vi "SMO.ByRefWithEvents.Process.vi"(8 "error in (no error)":errorcluster, 11 "SMO.ByRefWithEvents in":refnum<class "SMO.ByRefWithEvents.lvclass">) -> (0 "error out":errorcluster)   [LabVIEW 2013, in "SMO.ByRefWithEvents.lvclass"]
uses:
  SMO.ByRefWithEvents.lvclass
  <vilib>/JKI/JKI SMO/SMO/SMO.lvclass
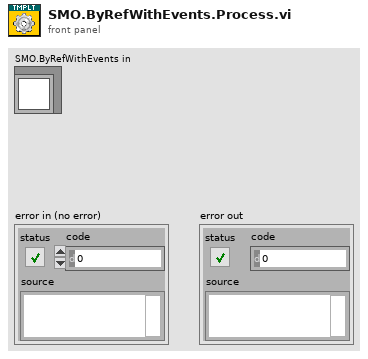
[diagram p1: front panel]
types:
  T1 = enum32{"invalid app kind", "Development System", "Run Time System", "Student Edition", "Embedded LabVIEW", "Evaluation", "Custom"}
  T2 = cluster{"Current VI Reference":refnum<vi>, "Close Panel on Exit?":bool, "error":errorcluster, "Standalone":bool}
  T3 = enum32{"Invalid", "Standard", "Closed", "Hidden", "Minimized", "Maximized"}
  T4 = cluster{"Core":cluster{"Current VI Reference":refnum<vi>, "Close Panel on Exit?":bool, "error":errorcluster, "Standalone":bool}, "Self Reference":refnum<class "SMO.ByRefWithEvents.lvclass">, "Your string data":string}
  T5 = typedef "SMO.lvclass/SMOState --Enum.ctl" = enum16{"unknown", "Created", "Started", "Stopped"}
  T6 = typedef "SMO.lvclass/Protected Events.ctl" = cluster{"StopProcesses":refnum<user-event>, "AbortProcesses":refnum<user-event>, "Config Changed":refnum<user-event>}
  T7 = typedef "SMO.ByRefWithEvents.lvclass/ProtectedEvents--Cluster.ctl" = cluster{"API_Template":refnum<user-event>}
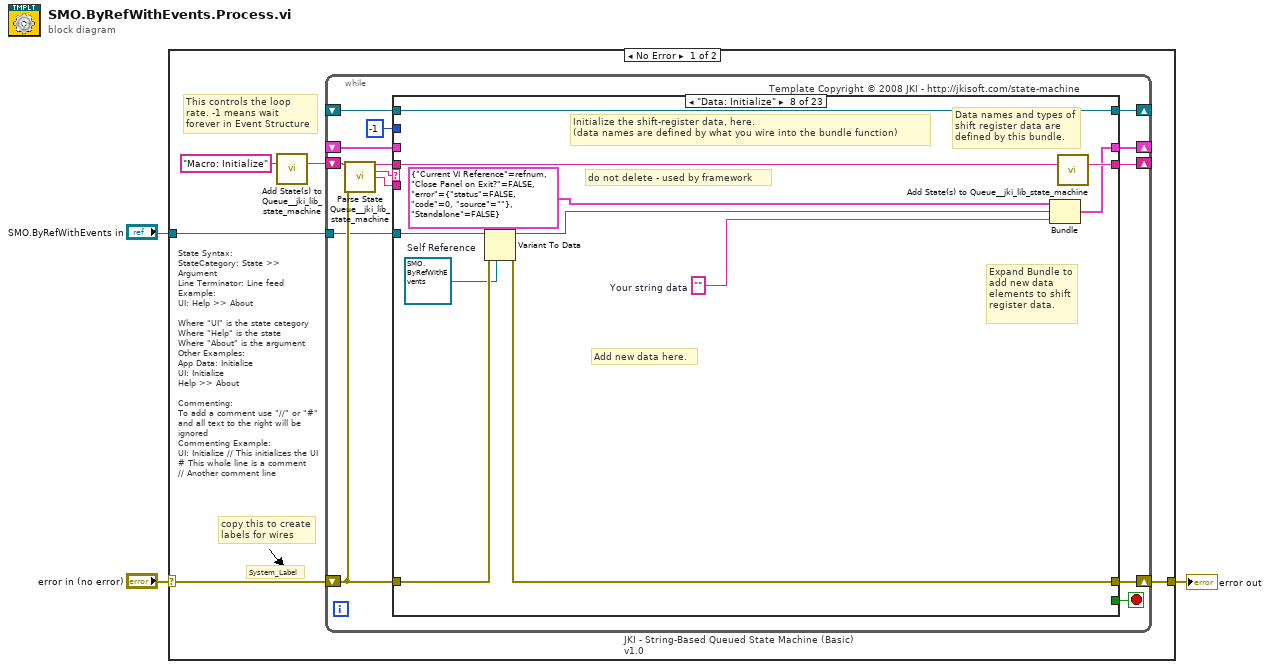
[diagram p0: block diagram]
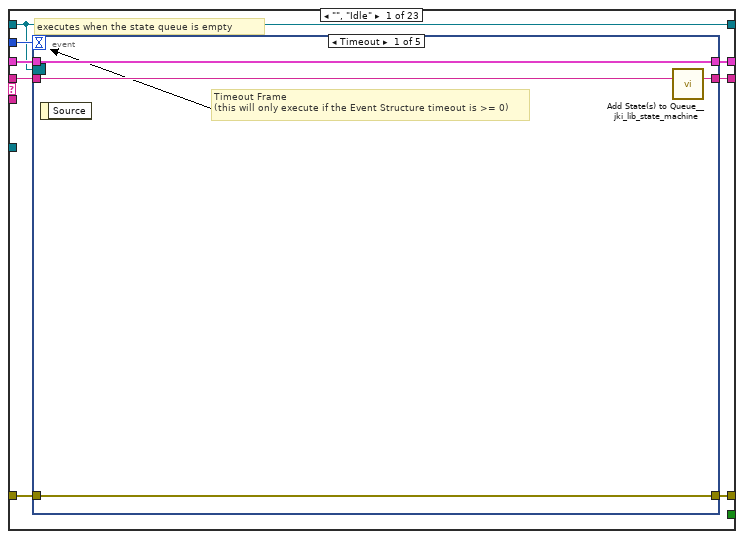
[diagram p2: hidden frame]
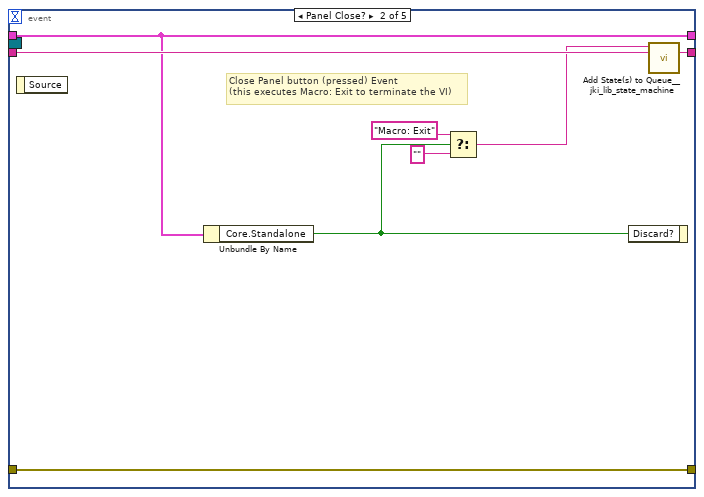
[diagram p3: hidden frame]
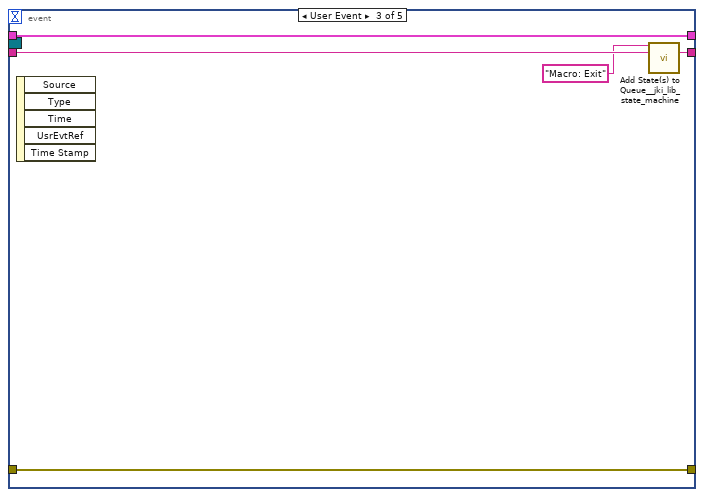
[diagram p4: hidden frame]
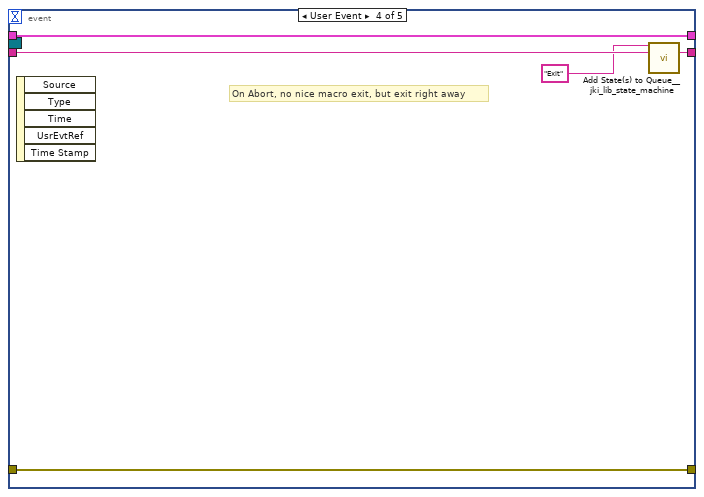
[diagram p5: hidden frame]
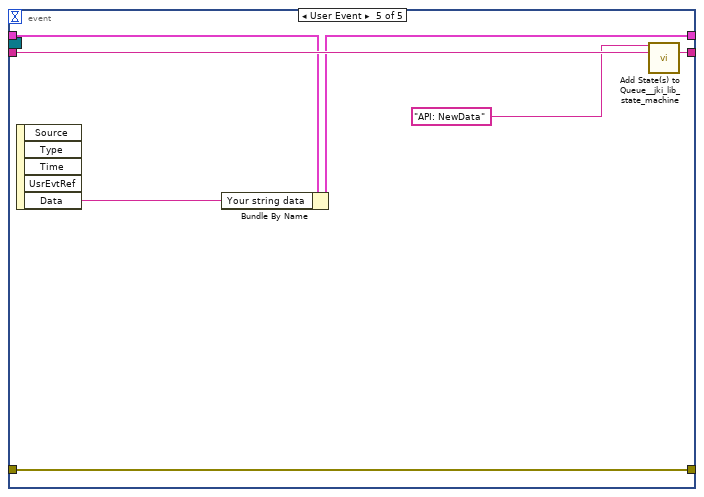
[diagram p6: hidden frame]
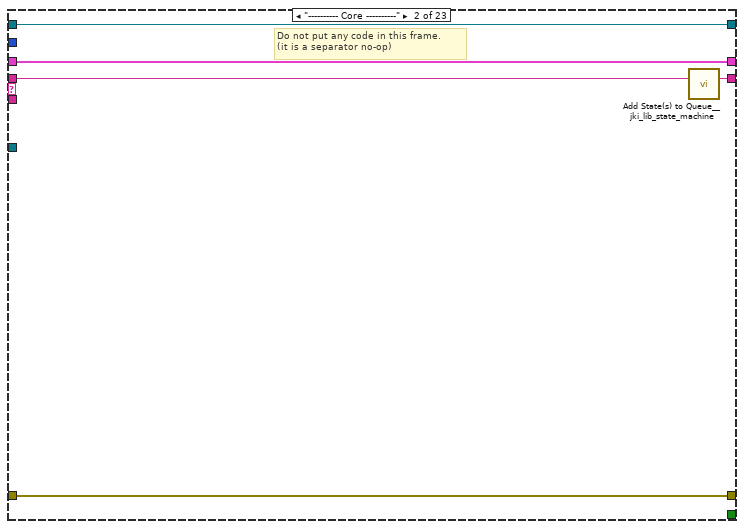
[diagram p7: hidden frame]
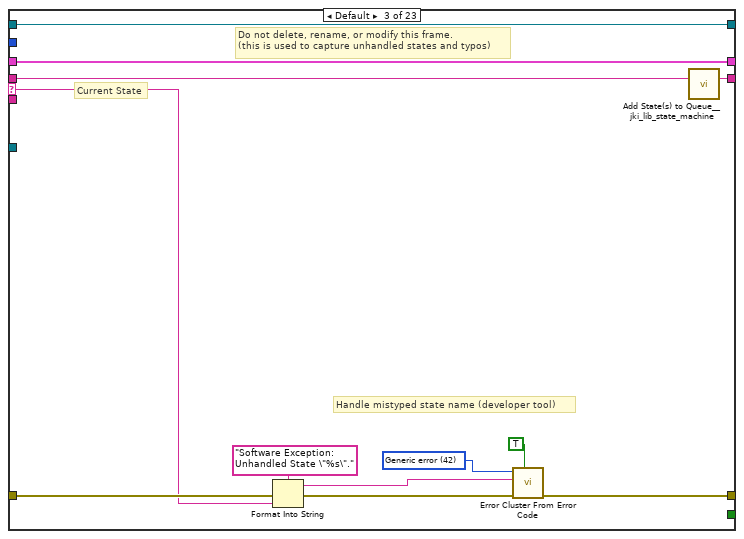
[diagram p8: hidden frame]
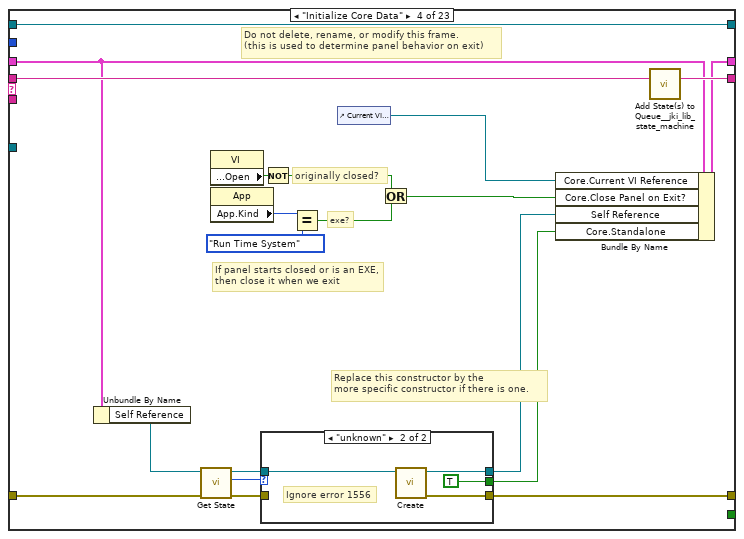
[diagram p9: hidden frame]
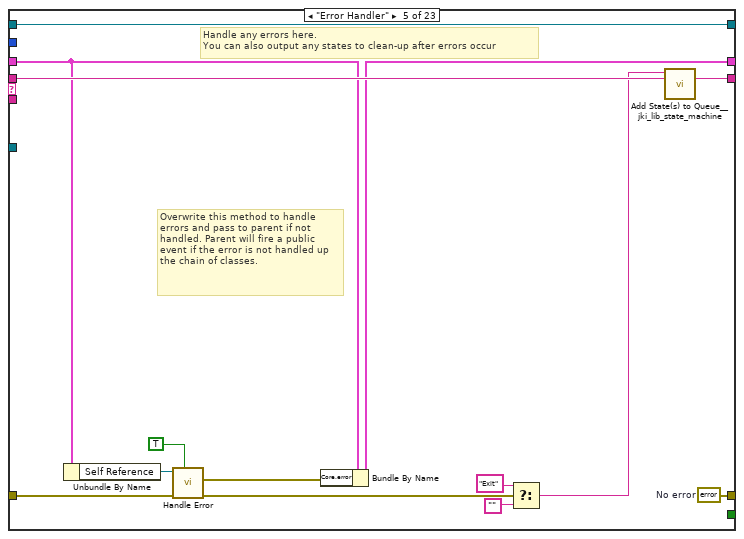
[diagram p11: hidden frame]
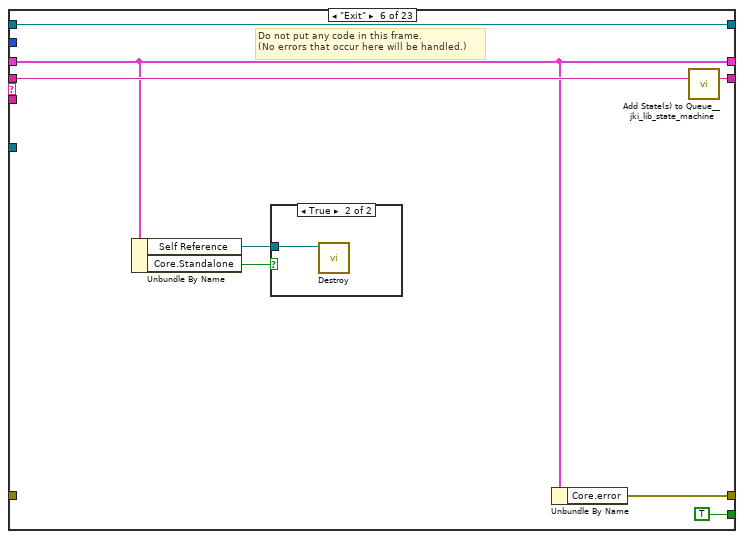
[diagram p12: hidden frame]
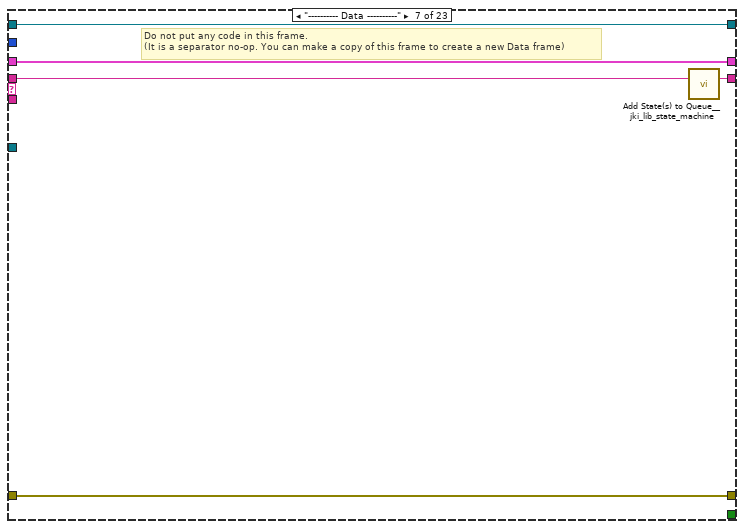
[diagram p14: hidden frame]
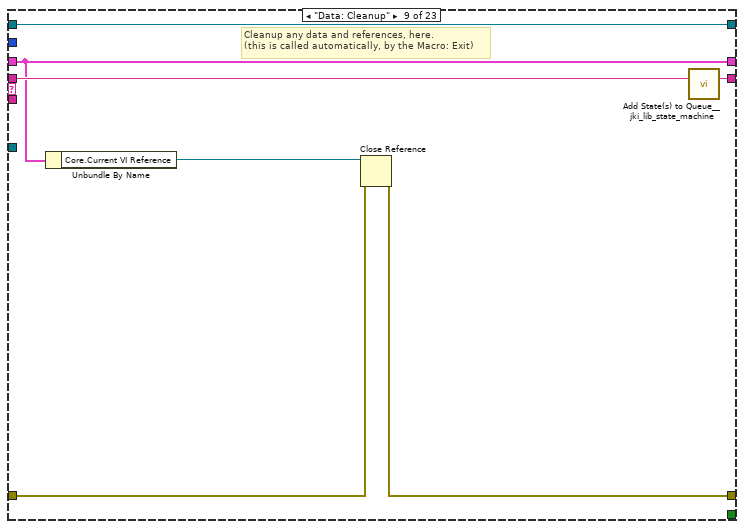
[diagram p15: hidden frame]
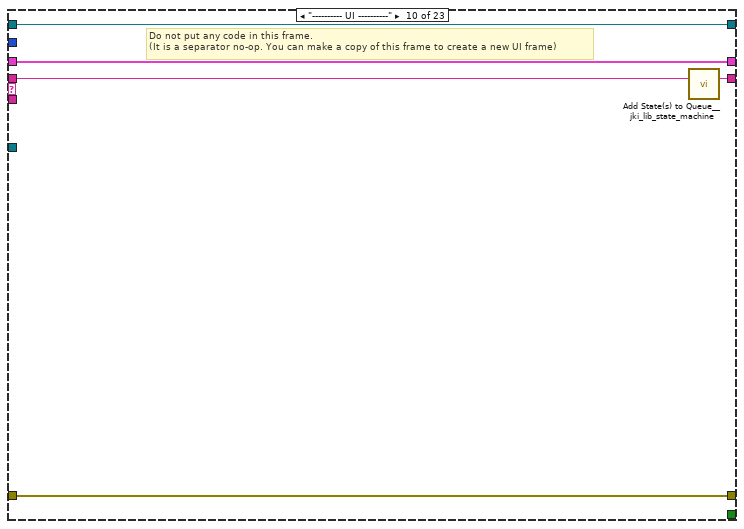
[diagram p16: hidden frame]
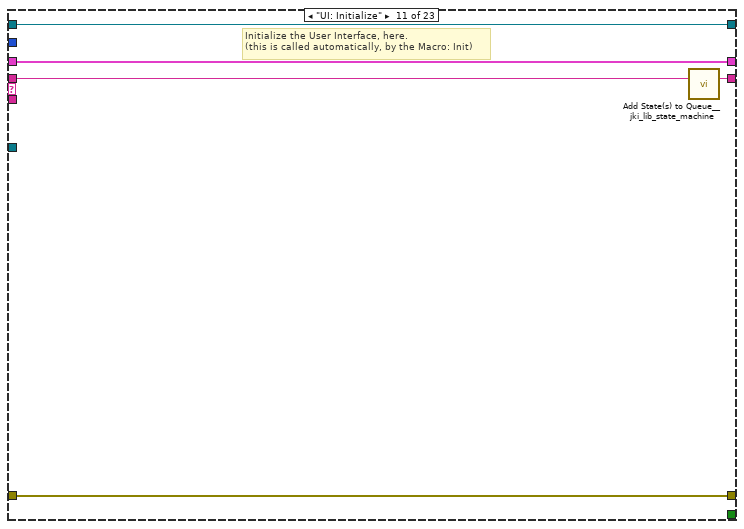
[diagram p17: hidden frame]
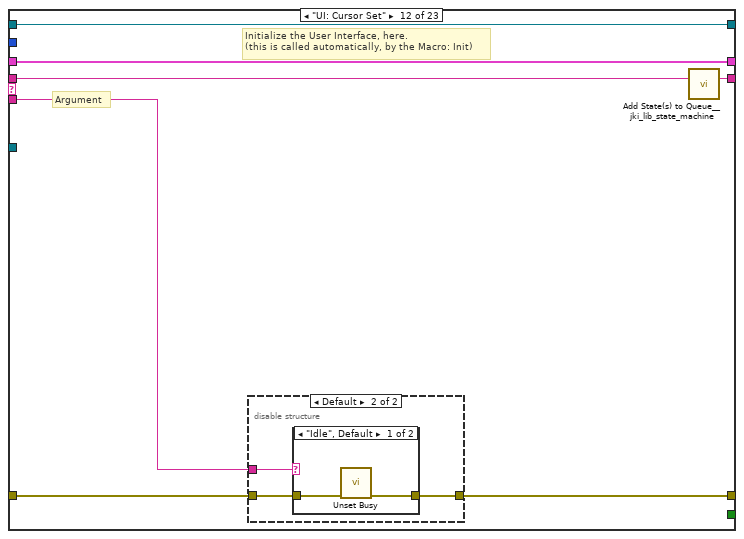
[diagram p18: hidden frame]
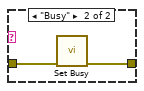
[diagram p20: hidden frame]
diagram:
  n1 = case shown="No Error" "error in (no error)" {
    selector: "error in (no error)" -> [w5 w290]
    tunnel: "SMO.ByRefWithEvents in" -> [w6 _]
    tunnel: [w4 w290] -> w3
    frame No Error {
      # "State Syntax:\nStateCategory: State >> Argument\nLine Terminator: Line feed\nExample:\nUI: Help >> About\n\nWhere \"UI\" is the state category\nWhere \"Help\" is the state\nWhere \"About\" is the argument\nOther Examples:\nApp Data: Initialize\nUI: Initialize\nHelp >> About\n\nCommenting:\nTo add a comment use \"//\" or \"#\" and all text to the right will be ignored\nCommenting Example:\nUI: Initialize // This initializes the UI\n# This whole line is a comment\n// Another comment line"
      # "copy this to create labels for wires"
      # "This controls the loop rate. -1 means wait forever in Event Structure"
      # "System_Label"
      n2 = call <vilib>:"Add State(s) to Queue__jki_lib_state_machine.vi"("State(s) in (\"\")"="Macro: Initialize") -> ("States Out"=w8:string)  [unwired: 14 in]
      n3 = while "JKI - String-Based Queued State Machine (Basic) v1.0" {
        shift-right: [w15] -> _
        shift-left: _ -> [w14]
        shift-right: [w18] -> w4
        shift-left: w5 -> [w12]
        shift-right: [w17] -> _
        shift-left: w8 -> [w19]
        tunnel: w6 -> [w11]
        shift-right: [w10] -> _
        shift-left: _ -> [w9]
        stop <- w16 stop-if-true
        # "Template Copyright © 2008 JKI - http://jkisoft.com/state-machine"
        n4 = call <vilib>:"Parse State Queue__jki_lib_state_machine.vi"("State Queue"=w19, "Error In (no error)"=w12) -> ("Remaining States"=w21:string, "Current State"=w22:string, "Arguments"=w20:string)  [unwired: 11 in]
        n5 = case shown="\"Data: Initialize\"" w22 {
          selector: w22 -> [_ _ w66 _ _ _ _ _ _ _ _ _ _ _ _ _ _ _ _ _ _ _ _]
          tunnel: w21 -> [w30 w64 w70 w96 w116 w124 w130 w141 w148 w153 w158 w165 w181 w213 w219 w230 w235 w244 w257 w270 w276 w281 w289]
          tunnel: w20 -> [_ _ _ _ _ _ _ _ _ _ _ w159 w175 _ _ _ _ _ _ _ _ _ _]
          tunnel: w14 -> [w28 w61 w68 w80 w105 w117 w127 _ w143 w150 w156 w163 w177 w210 w215 w221 w232 w241 w254 w268 w274 w279 w286]
          tunnel: [w27 w62 w72 w79 w107 w120 w128 w136 w144 w151 w155 w160 w178 w211 w217 w228 w233 w238 w255 w258 w272 w277 w282] -> w18
          tunnel: w12 -> [w26 w62 w71 w81 w112 _ w128 w137 w145 w151 w155 w161 w179 w211 w217 w228 w233 w239 w255 w262 w272 w277 w283]
          tunnel: [w29 w63 w69 w95 w115 w123 w129 w140 w147 w152 w157 w164 w180 w212 w218 w229 w234 w243 w256 w269 w275 w280 w288] -> w17
          tunnel: [_ _ _ _ _ TRUE _ _ _ _ _ _ _ _ _ _ _ _ _ _ _ _ _] -> w16
          tunnel: [w25 w61 w68 w94 w104 w117 w127 w139 w143 w150 w156 w163 w177 w210 w215 w221 w232 w241 w254 w268 w274 w279 w286] -> w15
          tunnel: -1 ("Timeout") -> [w24 _ _ _ _ _ _ _ _ _ _ _ _ _ _ _ _ _ _ _ _ _ _]
          tunnel: w11 -> [_ _ _ _ _ _ _ w134 _ _ _ _ _ _ _ _ _ _ _ _ _ _ _]
          tunnel: [w23 w60 w65 w87 w114 w121 w126 w132 w142 w149 w154 w162 w174 w209 w216 w222 w231 w242 w253 w267 w273 w278 w287] -> w10
          tunnel: w9 -> [w23 w60 w65 w87 w114 w121 w126 w132 w142 w149 w154 w162 w174 w209 w216 w222 w231 w242 w253 _ w273 w278 w287]
          frame "", "Idle" {
            # "executes when the state queue is empty"
            n6 = event shown="[0] Timeout" {
              selector: w23 -> [_ _ _ _ _]
              dyn-events: _ -> [_ _ _ _ _]
              timeout: w24 -> [_ _ _ _ _]
              tunnel: w30 -> [w34 w42 w47 w52 w59]
              tunnel: [w33 w41 w46 w51 w58] -> w29
              tunnel: w28 -> [w31 w37 w44 w49 w55]
              tunnel: [w32 w40 w45 w50 w57] -> w27
              tunnel: w26 -> [w32 w40 w45 w50 w57]
              tunnel: [w31 w37 w44 w49 w54] -> w25
              event Timeout {
                # "Timeout Frame\n(this will only execute if the Event Structure timeout is >= 0)"
                n7 = event-data() -> ()  [unwired: 1 in, 1 out]
                n8 = call <vilib>:"Add State(s) to Queue__jki_lib_state_machine.vi"("State(s) in (\"\")"=w34) -> ("States Out"=w33:string)  [unwired: 14 in]
              }
              event Panel Close? {
                # "Close Panel button (pressed) Event\n(this executes Macro: Exit to terminate the VI)"
                n9 = event-data() -> ()  [unwired: 1 in, 1 out]
                n10 = Unbundle By Name(w37) -> ("Core.Standalone"=w36:bool)
                n11 = Select(t="Macro: Exit", s=w36, f="") -> (s? t:f=w35:string)
                n12 = event-data("Discard?"=w36) -> ()  [unwired: 1 in, 1 out]
                n13 = call <vilib>:"Add State(s) to Queue__jki_lib_state_machine.vi"("State(s) in Front (\"\")"=w35, "State(s) in (\"\")"=w42) -> ("States Out"=w41:string)  [unwired: 13 in]
              }
              event User Event {
                n14 = event-data() -> ()  [unwired: 1 in, 5 out]
                n15 = call <vilib>:"Add State(s) to Queue__jki_lib_state_machine.vi"("State(s) in Front (\"\")"="Macro: Exit", "State(s) in (\"\")"=w47) -> ("States Out"=w46:string)  [unwired: 13 in]
              }
              event User Event {
                # "On Abort, no nice macro exit, but exit right away"
                n16 = event-data() -> ()  [unwired: 1 in, 5 out]
                n17 = call <vilib>:"Add State(s) to Queue__jki_lib_state_machine.vi"("State(s) in Front (\"\")"="Exit", "State(s) in (\"\")"=w52) -> ("States Out"=w51:string)  [unwired: 13 in]
              }
              event User Event {
                n18 = event-data() -> ("Data"=w56:string)  [unwired: 1 in, 4 out]
                n19 = Bundle By Name(cluster=w55, "Your string data"=w56) -> (w54:T4)
                n20 = call <vilib>:"Add State(s) to Queue__jki_lib_state_machine.vi"("State(s) in Front (\"\")"="API: NewData", "State(s) in (\"\")"=w59) -> ("States Out"=w58:string)  [unwired: 13 in]
              }
            }
          }
          frame "---------- Core ----------" {
            # "Do not put any code in this frame.\n(it is a separator no-op)"
            n21 = call <vilib>:"Add State(s) to Queue__jki_lib_state_machine.vi"("State(s) in (\"\")"=w64) -> ("States Out"=w63:string)  [unwired: 14 in]
          }
          frame Default {
            w75 = 42 items=["No error", "Argument error", "Memory is full", "Out of zone", "End of file", "File already open", "Generic file I/O error", "File not found", "File permission error", "Disk is full", "Duplicate path", "Too many files open", "System feature not enabled", "Resource file not found", "Cannot add resource", "Resource not found", "Image not found", "Image memory error", "Pen does not exist", "Config type invalid", "Config token not found", "Config parse error", "Config memory error", "Bad external code format", "Bad external code offset", "External code not present", "Null window", "Destroy window error", "Null menu", "Print aborted", "Bad print record", "Print driver error", "Windows error during printing", "Memory error during printing", "Print dialog error", "Generic print error", "Invalid device refnum", "Device not found", "Device parameter error", "Device unit error", "Cannot open device", "Device call aborted", "Generic error", "Cancelled by user", "Object ID too low", "Object ID too high", "Object not in heap", "Unknown heap", "Unknown object (invalid DefProc)", "Unknown object (DefProc not in table)", "Message out of range", "Invalid (null) method", "Unknown message", "Manager call not supported", "Bad address", "Network operation in progress", "Network operation timed out", "Connection is busy", "Network attribute not supported", "Network error", "Address in use", "System out of memory", "Connection aborted", "Connection refused", "Not connected", "Already connected", "Connection closed", "Initialization error (interapplication manager)", "Bad occurrence", "Wait on unbound occurrence handler", "Occurrence queue overflow", "Datalog type conflict", "Unused", "Unrecognized type (interapplication manager)", "Memory corrupt", "Failed to make temporary DLL", "Old CIN version", "Drag socket not found", "Failed to load drop-object", "Failed to register OLE object", "Failed to release OLE object", "Format specifier type mismatch", "Unknown format specifier", "Too few format specifiers", "Too many format specifiers", "Scan failed", "Newer CIN version", "Error converting to variant", "Runtime menu error", "Password tampered", "Variant attribute not found", "Incompatible variant data type", "Event data is not available", "Event Store is not present", "Occurrence is not found", "Event Queue is not created", "Event info is not available", "Refnum passed is NULL", "Error retrieving Class GUID", "Error retrieving CoClass GUID", "Error retrieving TypeLib GUID.", "Bad built application magic bytes.", "Specific driver is different from the specific driver associated with the Logical Name.", "There is no session opened to the class driver.", "Max Error", "MAX - Error with config objects", "MAX - Error loading configuration", "MAX - Group not supported"]
            # "Current State"
            # "Do not delete, rename, or modify this frame.\n(this is used to capture unhandled states and typos)"
            # "Handle mistyped state name (developer tool)"
            n22 = Format Into String(format string="Software Exception: Unhandled State \"%s\"." ("message"), error in=w71, w66) -> (resulting string=w74:string, error out=w73:errorcluster)  [unwired: 1 in]
            n23 = call <vilib>:"Error Cluster From Error Code.vi"("show call chain? (False)"=TRUE, "error in (no error)"=w73, "error message (\"\")"=w74, "error code (0)"=w75) -> ("error out"=w72:errorcluster)  [unwired: 5 in]
            n24 = call <vilib>:"Add State(s) to Queue__jki_lib_state_machine.vi"("State(s) in (\"\")"=w70) -> ("States Out"=w69:string)  [unwired: 14 in]
          }
          frame "Initialize Core Data" {
            # "Replace this constructor by the\nmore specific constructor if there is one."
            # "Do not delete, rename, or modify this frame.\n(this is used to determine panel behavior on exit)"
            # "originally closed?"
            # "exe?"
            # "If panel starts closed or is an EXE, then close it when we exit"
            n25 = Unbundle By Name(w80) -> ("Self Reference"=w85:refnum<class "SMO.ByRefWithEvents.lvclass">)
            n26 = call <vilib>:"Get State.vi"("error in (no error)"=w81, "SMO"=w85) -> ("error out"=w83:errorcluster, "SMO State"=w82:T5, "SMO out"=w84:refnum<class "SMO.ByRefWithEvents.lvclass">)  [unwired: 7 in]
            n27 = property class="VI"() -> ("Front Panel.Open"=w93:bool)  [unwired: 2 in, 2 out]
            n28 = property class="App"() -> ("App.Kind"=w92:T1)  [unwired: 2 in, 2 out]
            n29 = case shown="\"unknown\"" w82 {
              tunnel: w84 -> [w98 w102]
              tunnel: w83 -> [w97 _]
              tunnel: [w97 w101] -> w79
              tunnel: [w98 w100] -> w78
              tunnel: [_ TRUE] -> w77
              frame Default {
              }
              frame "unknown" {
                # "Ignore error 1556"
                n30 = call <vilib>:"Create.vi"("SMO"=w102) -> ("error out"=w101:errorcluster, "SMO out"=w100:refnum<class "SMO.ByRefWithEvents.lvclass">)  [unwired: 8 in, 1 out]
              }
            }
            n31 = Not(x=w93) -> (.not. x?=w90:bool)
            n32 = Equal?(x=w92, y=T1."Run Time System" ("Application:Kind")) -> (x = y?=w89:bool)
            n33 = control-ref of="Current VI Reference"() -> (w86:refnum<vi>)
            n34 = Or(x=w90, y=w89) -> (x .or. y?=w88:bool)
            n35 = Bundle By Name(cluster=w80, "Core.Current VI Reference"=w86, "Core.Close Panel on Exit?"=w88, "Self Reference"=w78, "Core.Standalone"=w77) -> (w94:T4)
            n36 = call <vilib>:"Add State(s) to Queue__jki_lib_state_machine.vi"("State(s) in (\"\")"=w96) -> ("States Out"=w95:string)  [unwired: 14 in]
          }
          frame "Error Handler" {
            w107 = errorcluster {"status"=FALSE, "code"=0, "source"=""}  # No error
            # "Overwrite this method to handle errors and pass to parent if not handled. Parent will fire a public event if the error is not handled up the chain of classes."
            # "Handle any errors here.\nYou can also output any states to clean-up after errors occur"
            n37 = Unbundle By Name(w105) -> ("Self Reference"=w113:refnum<class "SMO.ByRefWithEvents.lvclass">)
            n38 = call-dynamic "Handle Error.vi"("Stop on Unhandled Error (T)"=TRUE, "error in"=w112, "SMO"=w113) -> ("handling error"=w108:errorcluster, "Unhandled error"=w106:errorcluster)  [unwired: 6 in, 1 out]
            n39 = Bundle By Name(cluster=w105, "Core.error"=w106) -> (w104:T4)
            n40 = Select(t="Exit", s=w108, f="") -> (s? t:f=w109:string)
            n41 = call <vilib>:"Add State(s) to Queue__jki_lib_state_machine.vi"("State(s) in Front (\"\")"=w109, "State(s) in (\"\")"=w116) -> ("States Out"=w115:string)  [unwired: 13 in]
          }
          frame "Exit" {
            # "Do not put any code in this frame.\n(No errors that occur here will be handled.)"
            n42 = Unbundle By Name(w117) -> ("Self Reference"=w119:refnum<class "SMO.ByRefWithEvents.lvclass">, "Core.Standalone"=w118:bool)
            n43 = case shown="True" w118 {
              tunnel: w119 -> [_ w125]
              frame False {
              }
              frame True {
                n44 = call <vilib>:"Destroy.vi"("SMO"=w125) -> ()  [unwired: 10 in, 1 out]
              }
            }
            n45 = Unbundle By Name(w117) -> ("Core.error"=w120:errorcluster)
            n46 = call <vilib>:"Add State(s) to Queue__jki_lib_state_machine.vi"("State(s) in (\"\")"=w124) -> ("States Out"=w123:string)  [unwired: 14 in]
          }
          frame "---------- Data ----------" {
            # "Do not put any code in this frame.\n(It is a separator no-op. You can make a copy of this frame to create a new Data frame)"
            n47 = call <vilib>:"Add State(s) to Queue__jki_lib_state_machine.vi"("State(s) in (\"\")"=w130) -> ("States Out"=w129:string)  [unwired: 14 in]
          }
          frame "Data: Initialize" {
            w135 = refnum<class "SMO.ByRefWithEvents.lvclass"> refnum  # Self Reference
            w138 = ""  # Your string data
            # "do not delete - used by framework"
            # "Expand Bundle to add new data elements to shift register data."
            # "Add new data here."
            # "Data names and types of shift register data are defined by this bundle."
            # "Initialize the shift-register data, here.\n(data names are defined by what you wire into the bundle function)"
            n48 = Variant To Data(error in=w137, type=w135, Variant=w134) -> (data=w133:refnum<class "SMO.ByRefWithEvents.lvclass">, error out=w136:errorcluster)
            n49 = Bundle("Core"=T2 {"Current VI Reference"=refnum, "Close Panel on Exit?"=FALSE, "error"={"status"=FALSE, "code"=0, "source"=""}, "Standalone"=FALSE}, "Self Reference"=w133, "Your string data"=w138) -> (w139:T4)  [unwired: 1 in]
            n50 = call <vilib>:"Add State(s) to Queue__jki_lib_state_machine.vi"("State(s) in (\"\")"=w141) -> ("States Out"=w140:string)  [unwired: 14 in]
          }
          frame "Data: Cleanup" {
            # "Cleanup any data and references, here.\n(this is called automatically, by the Macro: Exit)"
            n51 = Unbundle By Name(w143) -> ("Core.Current VI Reference"=w146:refnum<vi>)
            n52 = Close Reference(reference=w146, error in (no error)=w145) -> (error out=w144:errorcluster)
            n53 = call <vilib>:"Add State(s) to Queue__jki_lib_state_machine.vi"("State(s) in (\"\")"=w148) -> ("States Out"=w147:string)  [unwired: 14 in]
          }
          frame "---------- UI ----------" {
            # "Do not put any code in this frame.\n(It is a separator no-op. You can make a copy of this frame to create a new UI frame)"
            n54 = call <vilib>:"Add State(s) to Queue__jki_lib_state_machine.vi"("State(s) in (\"\")"=w153) -> ("States Out"=w152:string)  [unwired: 14 in]
          }
          frame "UI: Initialize" {
            # "Initialize the User Interface, here.\n(this is called automatically, by the Macro: Init)"
            n55 = call <vilib>:"Add State(s) to Queue__jki_lib_state_machine.vi"("State(s) in (\"\")"=w158) -> ("States Out"=w157:string)  [unwired: 14 in]
          }
          frame "UI: Cursor Set" {
            # "Argument"
            # "Initialize the User Interface, here.\n(this is called automatically, by the Macro: Init)"
            n56 = disable-structure shown="Default" {
              disable-tunnel: w161 -> [w166 w169]
              disable-tunnel: [w166 w168] -> w160
              disable-tunnel: w159 -> [_ w167]
              frame condition #0 {
              }
              frame condition #1 (active) {
                n57 = case shown="\"Idle\", Default" w167 {
                  tunnel: w169 -> [w171 w173]
                  tunnel: [w170 w172] -> w168
                  frame "Idle", Default {
                    n58 = call <vilib>:"Unset Busy.vi"("error in (no error)"=w171) -> ("error out"=w170:errorcluster)  [unwired: 10 in]
                  }
                  frame "Busy" {
                    n59 = call <vilib>:"Set Busy.vi"("error in (no error)"=w173) -> ("error out"=w172:errorcluster)  [unwired: 9 in, 1 out]
                  }
                }
              }
            }
            n60 = call <vilib>:"Add State(s) to Queue__jki_lib_state_machine.vi"("State(s) in (\"\")"=w165) -> ("States Out"=w164:string)  [unwired: 14 in]
          }
          frame "UI: Front Panel State" {
            # "Argument"
            # "Set Front Panel Open or Closed\n(Usage: \"UI: Front Panel State >> Open|Close\")"
            n61 = Unbundle By Name(w177) -> ("Core.Current VI Reference"=w176:refnum<vi>)
            n62 = disable-structure shown="Default" {
              disable-tunnel: w179 -> [w185 w208]
              disable-tunnel: [w184 w208] -> w178
              disable-tunnel: w176 -> [w183 _]
              disable-tunnel: w175 -> [w182 _]
              frame condition #0 (active) {
                n63 = case shown="\"Close\"" w182 {
                  tunnel: w185 -> [w189 w202]
                  tunnel: [w191 w203] -> w184
                  tunnel: w183 -> [w190 w200]
                  frame "Open", Default {
                    n64 = property class="VI"(reference=w190, error in=w189) -> (reference out=w187:refnum<vi>, error out=w188:errorcluster, "FP.State"=w186:T3)
                    n65 = case shown="\"Closed\"" w186 {
                      tunnel: [w194 w197] -> w191
                      tunnel: w188 -> [w193 w197]
                      tunnel: w187 -> [w192 _]
                      frame "Closed" {
                        n66 = invoke class="VI" method="FP.Open"(reference=w192, error in=w193, "Activate"=TRUE, "State"=T3."Standard") -> (error out=w194:errorcluster)  [unwired: 1 in, 4 out]
                      }
                      frame Default {
                      }
                    }
                  }
                  frame "Close" {
                    n67 = property class="VI"(reference=w200, error in=w202) -> (reference out=w199:refnum<vi>, error out=w201:errorcluster, "FP.State"=w198:T3)
                    n68 = case shown="Default" w198 {
                      tunnel: [w204 w207] -> w203
                      tunnel: w201 -> [w204 w206]
                      tunnel: w199 -> [_ w205]
                      frame "Invalid", "Closed" {
                      }
                      frame Default {
                        n69 = invoke class="VI" method="FP.Close"(reference=w205, error in=w206) -> (error out=w207:errorcluster)  [unwired: 1 in, 2 out]
                      }
                    }
                  }
                }
              }
              frame condition #1 {
              }
            }
            n70 = call <vilib>:"Add State(s) to Queue__jki_lib_state_machine.vi"("State(s) in (\"\")"=w181) -> ("States Out"=w180:string)  [unwired: 14 in]
          }
          frame "---------- Macro ----------" {
            # "Do not put any code in this frame.\n(It is a separator no-op. You can make a copy of this frame to create a new Macro frame)"
            n71 = call <vilib>:"Add State(s) to Queue__jki_lib_state_machine.vi"("State(s) in (\"\")"=w213) -> ("States Out"=w212:string)  [unwired: 14 in]
          }
          frame "Macro: Initialize" {
            # "Initialization Macro\n(This is called once, when the VI starts)"
            n72 = call <vilib>:"Add State(s) to Queue__jki_lib_state_machine.vi"("State(s) in Front (\"\")"="Data: Initialize\nInitialize Core Data\nEvents: Register\nProcess: Sync", "State(s) in (\"\")"=w219) -> ("States Out"=w218:string)  [unwired: 13 in]
          }
          frame "Macro: Exit" {
            # "Exit Macro\n(This is called once, when the VI exits)"
            n73 = Unbundle By Name(w221) -> ("Core.Close Panel on Exit?"=w227:bool)
            n74 = Select(t="UI: Front Panel State >> Close", s=w227, f="") -> (s? t:f=w224:string)
            n75 = call <vilib>:"Add State(s) to Queue__jki_lib_state_machine.vi"("State(s) in (\"\")"=w224, "State(s) at Back (\"\")"="Data: Cleanup\nEvents: Unregister\nProcess: Sync\nExit") -> ("States Out"=w223:string)  [unwired: 13 in]
            n76 = call <vilib>:"Add State(s) to Queue__jki_lib_state_machine.vi"("State(s) in Front (\"\")"=w223, "State(s) in (\"\")"=w230) -> ("States Out"=w229:string)  [unwired: 13 in]
          }
          frame "---------- Process ----------" {
            # "Template Separator\n(You can make a copy of, or modify, this frame)"
            n77 = call <vilib>:"Add State(s) to Queue__jki_lib_state_machine.vi"("State(s) in (\"\")"=w235) -> ("States Out"=w234:string)  [unwired: 14 in]
          }
          frame "Process: Sync" {
            n78 = Unbundle By Name(w241) -> ("Self Reference"=w240:refnum<class "SMO.ByRefWithEvents.lvclass">, "Core.Standalone"=w236:bool)
            n79 = case shown="False" w236 {
              tunnel: w240 -> [w248 _]
              tunnel: w239 -> [w247 w252]
              tunnel: [w246 w252] -> w238
              tunnel: [w245 _] -> w237
              frame False {
                n80 = call <vilib>:"WaitOnProcessSync.vi"("error in (no error)"=w247, "SMO"=w248) -> ("error out"=w246:errorcluster, "Don't run?"=w251:bool)  [unwired: 7 in, 1 out]
                n81 = Select(t="Data: Cleanup\nEvents: Unregister\nExit", s=w251, f="") -> (s? t:f=w245:string)
              }
              frame True {
              }
            }
            n82 = call <vilib>:"Add State(s) to Queue__jki_lib_state_machine.vi"("State(s) in Front (\"\")"=w237, "State(s) in (\"\")"=w244) -> ("States Out"=w243:string)  [unwired: 13 in]
          }
          frame "---------- Events ----------" {
            # "Template Separator\n(You can make a copy of, or modify, this frame)"
            n83 = call <vilib>:"Add State(s) to Queue__jki_lib_state_machine.vi"("State(s) in (\"\")"=w257) -> ("States Out"=w256:string)  [unwired: 14 in]
          }
          frame "Events: Register" {
            # "Expand to add\nmore events"
            # "Self Events (API Calls)"
            # "Base Class Protected Events"
            n84 = Unbundle By Name(w268) -> ("Self Reference"=w263:refnum<class "SMO.ByRefWithEvents.lvclass">)
            n85 = call <vilib>:"GetProtectedEvents.vi"("SMO"=w263) -> ("error out"=w259:errorcluster, "SMO Protected Events"=w266:T6, "SMO out"=w265:refnum<class "SMO.ByRefWithEvents.lvclass">)  [unwired: 8 in]
            n86 = call "SMO.ByRefWithEvents.GetProtectedEvents.vi"("SMO.ByRefWithEvents"=w265) -> ("error out"=w260:errorcluster, "Protected Events"=w264:T7)  [unwired: 8 in, 1 out]
            n87 = register-events(w266, w264) -> (reference out=w267:refnum<event-registration>, error out=w261:errorcluster)  [unwired: 2 in]
            n88 = Merge Errors(w262, w261, w260, w259) -> (w258:errorcluster)
            n89 = call <vilib>:"Add State(s) to Queue__jki_lib_state_machine.vi"("State(s) in (\"\")"=w270) -> ("States Out"=w269:string)  [unwired: 14 in]
          }
          frame "Events: Unregister" {
            n90 = Unregister For Events(event registration refnum=w273, error in=w272) -> (error out=w271:errorcluster)
            n91 = call <vilib>:"Clear Errors.vi"("error in (no error)"=w271) -> ()  [unwired: 6 in, 1 out]
            n92 = call <vilib>:"Add State(s) to Queue__jki_lib_state_machine.vi"("State(s) in (\"\")"=w276) -> ("States Out"=w275:string)  [unwired: 14 in]
          }
          frame "---------- API ----------" {
            n93 = call <vilib>:"Add State(s) to Queue__jki_lib_state_machine.vi"("State(s) in (\"\")"=w281) -> ("States Out"=w280:string)  [unwired: 14 in]
          }
          frame "API: NewData" {
            n94 = Unbundle By Name(w286) -> ("Self Reference"=w285:refnum<class "SMO.ByRefWithEvents.lvclass">, "Your string data"=w284:string)
            n95 = call "SMO.ByRefWithEvents.SetData.vi"("error in (no error)"=w283, "Data In"=w284, "SMO.ByRefWithEvents"=w285) -> ("error out"=w282:errorcluster)  [unwired: 7 in, 1 out]
            n96 = call <vilib>:"Add State(s) to Queue__jki_lib_state_machine.vi"("State(s) in (\"\")"=w289) -> ("States Out"=w288:string)  [unwired: 14 in]
          }
        }
      }
    }
    frame Error {
    }
  }
  "error out" <- w3
